vi "Add New Data Array.vi"(8 "error in (no error)":errorcluster, 11 "Node Ptr":u64 format="%.0x") -> (0 "error out":errorcluster)   [LabVIEW 2018, in "Instrument Addon System Explorer.lvlib"]
uses:
  Instrument Addon System Explorer.lvlib
  Addon Shared/Types/FG Control.ctl
  Addon Shared/Types/Data Parameters.ctl
  Addon Shared/Types/Protocol Data Type.ctl
  Addon Shared/Types/Data Channel Type.ctl
  Addon Shared/Types/Type Cast Type.ctl
  Addon Shared/Types/Endian.ctl
  Addon Shared/SubVIs/Constants.vi
  <vilib>/NI Veristand/Custom Device API/NI VeriStand - Get Item Property.vi
  <vilib>/NI Veristand/Custom Device API/Get Item Property (U32).vi
  <vilib>/NI Veristand/Custom Device API/Get Item Property (String).vi
  <vilib>/NI Veristand/Custom Device API/Get Item Property (String Array).vi
  <vilib>/NI Veristand/Custom Device API/Set Item Property (U32).vi
  <vilib>/NI Veristand/Custom Device API/Set Item Property (String).vi
  <vilib>/NI Veristand/Custom Device API/Set Item Property (String Array).vi
  <vilib>/NI Veristand/Custom Device API/NI VeriStand - Set Custom Device Channel Value Table.vi
  <vilib>/NI Veristand/Custom Device API/NI VeriStand - Get Item Children.vi
  <vilib>/NI Veristand/Custom Device API/Custom Device API.lvlib
  Addon Shared/Instrument Addon Shared.lvlib
panel:
  in  "Tag":string
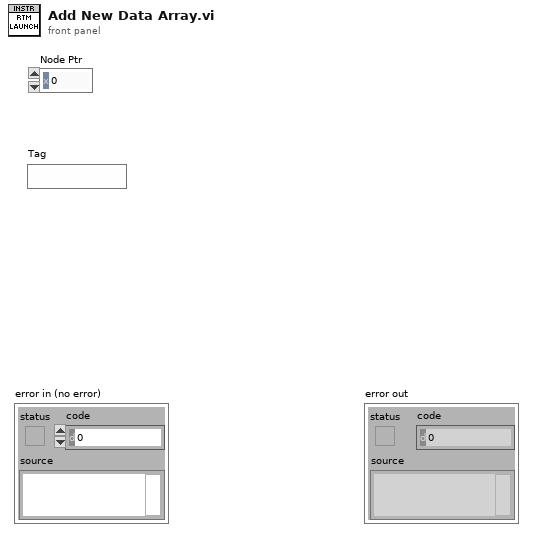
[diagram p1: front panel]
types:
  T1 = typedef "Instrument Addon Shared.lvlib/Data Parameters.ctl" = cluster{"Data Type":T2, "Channel Type":T3, "Format String":string, "Expected String":string, "Type":T4, "List":string[], "Delimiter":string, "Endian":T5}
  T2 = typedef "Instrument Addon Shared.lvlib/Protocol Data Type.ctl" = enum16{"Single Channel", "Array"}
  T3 = typedef "Instrument Addon Shared.lvlib/Data Channel Type.ctl" = enum16{"Format", "Comparison", "Type Cast", "Enumerated List"}
  T4 = typedef "Instrument Addon Shared.lvlib/Type Cast Type.ctl" = enum16{"DBL", "SGL", "U64", "U32", "U16", "U8", "I64", "I32", "I16", "I8"}
  T5 = typedef "Instrument Addon Shared.lvlib/Endian.ctl" = enum16{"Native", "Little", "Big"}
  T6 = typedef "Instrument Addon Shared.lvlib/FG Control.ctl" = enum16{"Get", "Set"}
  T7 = typedef "Custom Device API.lvlib/Custom Device Item Ref.ctl" = u64
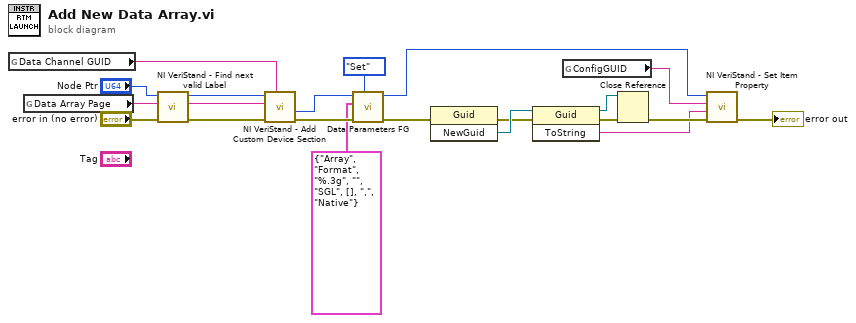
[diagram p0: block diagram]
diagram:
  n1 = global read "Constants.vi" "Data Channel GUID"() -> (w15:string)
  n2 = global read "Constants.vi" "Data Array Page"() -> (w19:string)
  n3 = call <vilib>:"NI VeriStand - Find next valid Label.vi"("error in (no error)"="error in (no error)", "Label"=w19, "Item Ref in"="Node Ptr") -> ("error out"=w16:errorcluster, "Label out"=w17:string, "Item Ref out"=w18:T7)  [unwired: 4 in, 2 out]
  n4 = call <vilib>:"NI VeriStand - Add Custom Device Section.vi"("GUID (Default Section)"=w15, "error in (no error)"=w16, "Section Name"=w17, "Parent Ref in"=w18) -> ("error out"=w6:errorcluster, "Section Ptr"=w4:T7)  [unwired: 4 in, 2 out]
  n5 = call "Data Parameters FG.vi"("Action"=FG_Control."Set", "error in (no error)"=w6, "Data Parameters"=T1 {"Data Type"=enum."Array", "Channel Type"=enum."Format", "Format String"="%.3g", "Expected String"="", "Type"=enum."SGL", "List"=[], "Delimiter"=",", "Endian"=enum."Native"}, "Item Ref in"=w4) -> ("error out"=w5:errorcluster, "Item Ref out"=w3:T7)  [unwired: 5 in, 1 out]
  n6 = invoke class="Guid" method="NewGuid"(error in=w5) -> (error out=w11:errorcluster, "NewGuid"=w12:refnum<k24>)  [unwired: 2 in, 1 out]
  n7 = invoke class="Guid" method="ToString"(reference=w12, error in=w11) -> (reference out=w13:refnum<k24>, error out=w10:errorcluster, "ToString"=w7:string)  [unwired: 1 in]
  n8 = global read "Constants.vi" "ConfigGUID"() -> (w14:string)
  n9 = Close Reference(reference=w13, error in (no error)=w10) -> (error out=w9:errorcluster)
  n10 = call-poly <vilib>:"NI VeriStand - Set Item Property.vi"("error in (no error)"=w9, "Value"=w7, "Property Name"=w14, "Item Ref in"=w3) -> ("error out"=→"error out":errorcluster)  [unwired: 5 in, 2 out]
